vi "WriteSpectroMeter.vi"(1 "本次文件名":string) -> ()   [LabVIEW 2018]
uses:
  Init/AllPath.vi
  Reslut.vi
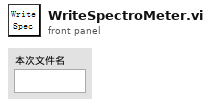
[diagram p1: front panel]
types:
  T1 = cluster{"光谱波形":cluster{"X":dbl[], "Y":dbl[]}, "中心波长":string, " 谱宽":string, " 中心波长Uint":string, " 谱宽 Uint":string}
  T2 = cluster{"能量/功率":path, " 示波器":path, " 光谱仪":path, "偏振":path, "近远场":cluster{" 近场图片":path, " 远场图片":path, "发散角数据":path}, "参数":path, " 基路径":path, "文件名信息":path}
  T3 = cluster{"激光器型号":string, "X":dbl, "Y":dbl, "Z":dbl, "Rotate":dbl, "Pitching":dbl, "DivergeAngle":dbl}
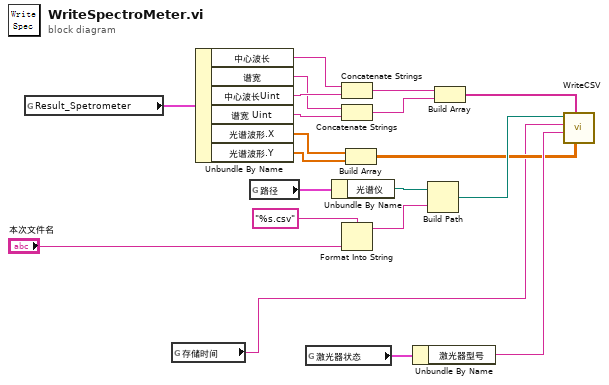
[diagram p0: block diagram]
diagram:
  n1 = global read "Reslut.vi" "Result_Spetrometer"() -> (w17:T1)
  n2 = global read "Reslut.vi" "存储时间"() -> (w1:string)
  n3 = Unbundle By Name(w17) -> ("中心波长"=w13:string, "谱宽"=w11:string, "中心波长Uint"=w12:string, "谱宽 Uint"=w10:string, "光谱波形.X"=w4:dbl[], "光谱波形.Y"=w3:dbl[])
  n4 = global read "AllPath.vi" "路径"() -> (w20:T2)
  n5 = global read "参数.vi" "激光器状态"() -> (w18:T3)
  n6 = Unbundle By Name(w20) -> ("光谱仪"=w19:path)
  n7 = Concatenate Strings(w13, w12) -> (w7:string)
  n8 = Concatenate Strings(w11, w10) -> (w6:string)
  n9 = Format Into String(format string="%s.csv" ("格式字符串"), "本次文件名") -> (resulting string=w14:string)  [unwired: 2 in, 1 out]
  n10 = Build Array(w4, w3) -> (w2:dbl[][])
  n11 = Unbundle By Name(w18) -> ("激光器型号"=w9:string)
  n12 = Build Path(base path=w19, name or relative path=w14) -> (appended path=w8:path)
  n13 = Build Array(w7, w6) -> (w5:string[])
  n14 = call "WriteCSV.vi"("波形"=w2, "通用数据"=w5, "任务编号"=w9, "时间"=w1, "file path (dialog if empty)"=w8) -> ()  [unwired: 7 in]
